vi "HexToString.vi"(1 "StrIn":string) -> (0 "StrOut":string)   [LabVIEW 2013]
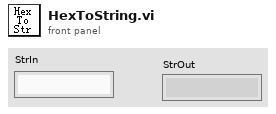
[diagram p1: front panel]
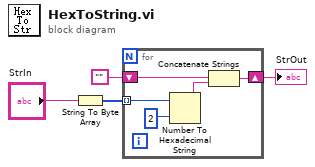
[diagram p0: block diagram]
diagram:
  n1 = String To Byte Array(string="StrIn") -> (unsigned byte array=w3:u8[])
  n2 = for {
    tunnel: w3 -> [w9] mode=indexing
    shift-right: [w6] -> w1
    shift-left: "" -> [w5]
    n3 = Number To Hexadecimal String(1:2, 2:w9) -> (0:w7:string)
    n4 = Concatenate Strings(w5, w7) -> (w6:string)
  }
  "StrOut" <- w1
